vi "4155C Apply Stress.vi"(2 "error in (no error)":errorcluster, 3 "Duration":dbl min=-100.0 max=100.0 format="%.2f", 4 "Emergency Stop":refnum<vi>, 5 "VISA resource name in":refnum<visa-resource-name>) -> (0 "error out":errorcluster, 1 "VISA Resource Name out":refnum<visa-resource-name>)   [LabVIEW 2019]
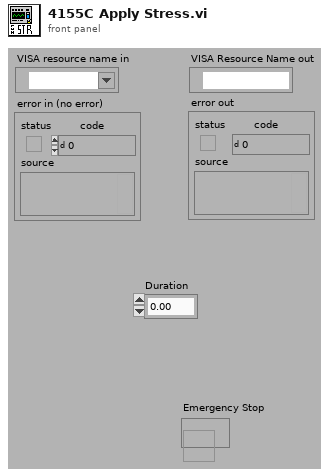
[diagram p1: front panel]
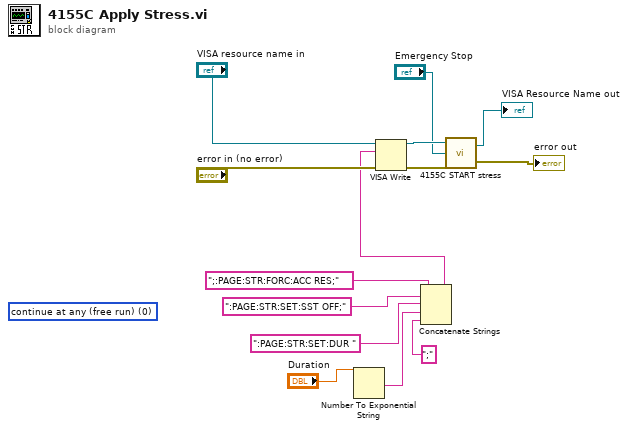
[diagram p0: block diagram]
diagram:
  (unwired) u8 0 items=["continue at any (free run)", "stop at any abnorm", "stop at compliance"] ("stop condition (free run:0)")
  n1 = Number To Exponential String(number="Duration") -> (E-format string=w12:string)  [unwired: 3 in]
  n2 = Concatenate Strings(";:PAGE:STR:FORC:ACC RES;" ("write buffer (\"\")"), ":PAGE:STR:SET:SST OFF;" ("write buffer (\"\")"), ":PAGE:STR:SET:DUR " ("write buffer (\"\")"), w12, ";" ("Substring")) -> (w9:string)
  n3 = VISA Write(VISA resource name="VISA resource name in", write buffer=w9, error in (no error)="error in (no error)") -> (VISA resource name out=w4:refnum<visa-resource-name>, error out=w6:errorcluster)  [unwired: 1 out]
  n4 = call "4155C START stress.vi"("error in (no error)"=w6, "Emergency Stop"="Emergency Stop", "VISA resource name in"=w4) -> ("error out"=→"error out":errorcluster, "VISA Resource Name out"=→"VISA Resource Name out":refnum<visa-resource-name>)
